vi "Subvi pixelclock start stop.vi"(1 "Nlines per frame":u16, 2 "Nlines per frame plus skips":u16, 3 "Nlines all":u16, 7 "Pixelclock/Lineclock":T1, 12 "Pixel_clock_trigger":bool) -> (4 "Gated pixelclock change":bool, 6 "Framegate":bool, 10 "Gated frameclock":bool)   [LabVIEW 2017]
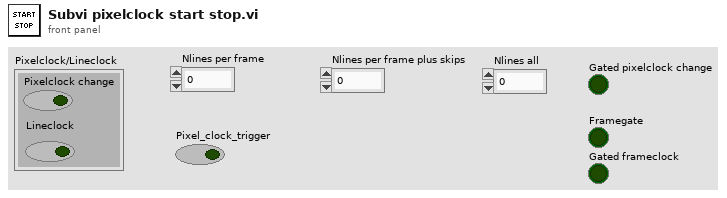
[diagram p1: front panel]
types:
  T1 = cluster{"Pixelclock change":bool, "Lineclock":bool}
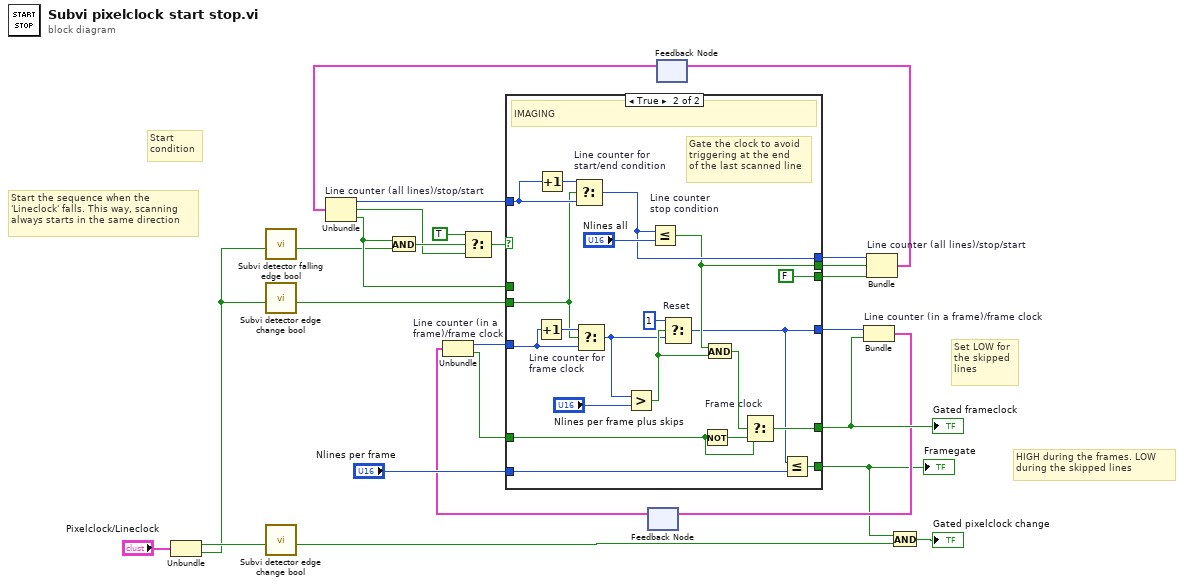
[diagram p0: block diagram]
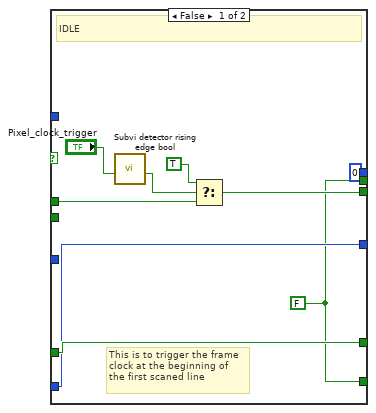
[diagram p2: hidden frame]
diagram:
  # "Set LOW for\nthe skipped\nlines"
  # "Start the sequence when the\n'Lineclock' falls. This way, scanning\nalways starts in the same direction"
  # "HIGH during the frames. LOW\nduring the skipped lines"
  # "Start\ncondition"
  n1 = Unbundle("Pixelclock/Lineclock") -> ("Pixelclock change"=w16:bool, "Lineclock"=w13:bool)
  n2 = call "Subvi detector falling edge bool.vi"("Input"=w13) -> ("Output"=w18:bool)  [unwired: 10 in]
  n3 = call "Subvi detector edge change bool.vi"("Input"=w13) -> ("Output"=w12:bool)  [unwired: 8 in]
  n4 = call "Subvi detector edge change bool.vi"("Input"=w16) -> ("Output"=w1:bool)  [unwired: 8 in]
  n5 = feedback #1() -> (w6:cluster{"Nlines per frame":u16, bool})  [unwired: 1 in]
  n6 = Unbundle "Line counter (in a frame)/frame clock"(w6) -> ("Nlines per frame"=w4:u16, w5:bool)
  n7 = feedback #2() -> (w26:cluster{u16, bool, bool})  [unwired: 1 in]
  n8 = Unbundle "Line counter (all lines)/stop/start"(w26) -> (w23:u16, w15:bool, w19:bool)
  n9 = And(x=w19, y=w18) -> (x .and. y?=w20:bool)
  n10 = Select(t=TRUE, s=w20, f=w15) -> (s? t:f=w22:bool)
  n11 = case shown="True" w22 {
    tunnel: w23 -> [_ w46]
    tunnel: [u16 0 w45] -> w24
    tunnel: [w31 FALSE] -> w21
    tunnel: w19 -> [w30 _]
    tunnel: [w29 w50] -> w8
    tunnel: w5 -> [w29 w49]
    tunnel: "Nlines per frame" -> [w28 w42]
    tunnel: [w28 w36] -> w9
    tunnel: w4 -> [_ w48]
    tunnel: w12 -> [_ w44]
    tunnel: [w27 w37] -> w2
    tunnel: [w27 w38] -> w10
    frame False {
      w27 = FALSE
      # "This is to trigger the frame\nclock at the beginning of\nthe first scaned line"
      # "IDLE"
      n12 = call "Subvi detector rising edge bool.vi"("Input"="Pixel_clock_trigger") -> ("Output"=w32:bool)  [unwired: 10 in]
      n13 = Select(t=TRUE, s=w32, f=w30) -> (s? t:f=w31:bool)
    }
    frame True {
      # "Gate the clock to avoid\ntriggering at the end\nof the last scanned line"
      # "IMAGING"
      n14 = Increment(x=w48) -> (x+1=w52:u16)
      n15 = Increment(x=w46) -> (x+1=w55:u16)
      n16 = Select "Line counter for\nstart/end condition"(t=w55, s=w44, f=w46) -> (s? t:f=w45:u16)
      n17 = Select "Line counter for\nframe clock"(t=w52, s=w44, f=w48) -> (s? t:f=w40:u16)
      n18 = Greater?(x=w40, y="Nlines per frame plus skips") -> (0:w41:bool)
      n19 = Less Or Equal? "Line counter\nstop condition"(x=w45, y="Nlines all") -> (x <= y?=w38:bool)
      n20 = Select "Reset"(t=u16 1, s=w41, f=w40) -> (s? t:f=w36:u16)
      n21 = Not(x=w49) -> (.not. x?=w53:bool)
      n22 = And(x=w38, y=w41) -> (x .and. y?=w43:bool)
      n23 = Select "Frame clock"(t=w53, s=w43, f=w49) -> (s? t:f=w50:bool)
      n24 = Less Or Equal?(x=w36, y=w42) -> (x <= y?=w37:bool)
    }
  }
  "Framegate" <- w2
  "Gated frameclock" <- w8
  n25 = Bundle "Line counter (in a frame)/frame clock"("Nlines per frame"=w9, w8) -> (w7:cluster{"Nlines per frame":u16, bool})  [unwired: 1 in]
  n26 = feedback-in #1(w7) -> ()
  n27 = Bundle "Line counter (all lines)/stop/start"(w24, w10, w21) -> (w11:cluster{u16, bool, bool})  [unwired: 1 in]
  n28 = feedback-in #2(w11) -> ()
  n29 = And(x=w2, y=w1) -> (x .and. y?=→"Gated pixelclock change":bool)
